vi "Write Current Filter.vi"(8 "error in (no error)":errorcluster, 10 "Current Filter":string, 11 "Filter_Wheel in":refnum<class "Filter_Wheel.lvclass">) -> (0 "error out":errorcluster, 3 "Filter_Wheel out":refnum<class "Filter_Wheel.lvclass">)   [LabVIEW 2018, in "Filter_Wheel.lvclass"]
uses:
  Filter_Wheel.lvclass
  Filter_Wheel.lvclass/Filter_Wheel.ctl
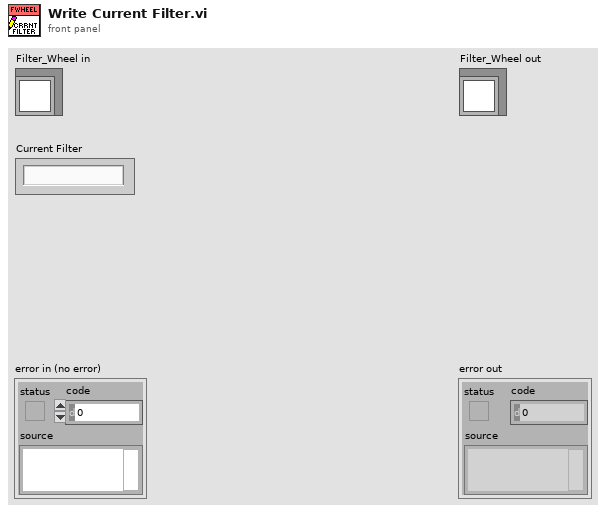
[diagram p1: front panel]
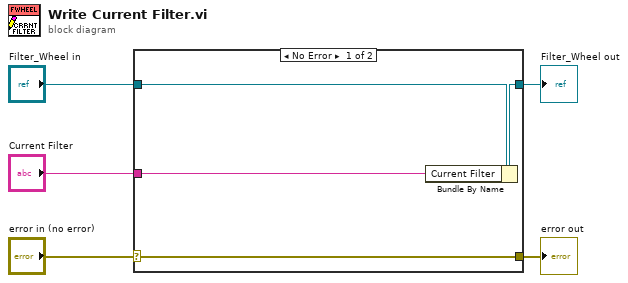
[diagram p0: block diagram]
diagram:
  n1 = case shown="No Error" "error in (no error)" {
    selector: "error in (no error)" -> [w9 w10]
    tunnel: [w9 w10] -> w4
    tunnel: [w7 w11] -> w2
    tunnel: "Filter_Wheel in" -> [w8 w11]
    tunnel: "Current Filter" -> [w6 _]
    frame No Error {
      n2 = Bundle By Name(cluster=w8, "Current Filter"=w6) -> (w7:refnum<class "Filter_Wheel.lvclass">)
    }
    frame Error {
    }
  }
  "error out" <- w4
  "Filter_Wheel out" <- w2
